vi "Read Locale.vi"(11 "MsgSerializer":refnum<class "MsgSerializer.lvclass">) -> (2 "Locale":string, 3 "MsgSerializer":refnum<class "MsgSerializer.lvclass">)   [LabVIEW 2013, in "Caraya.lvlib" / "MsgSerializer.lvclass"]
uses:
  MsgSerializer/MsgSerializer.lvclass
  MsgSerializer/MsgSerializer.lvclass/MsgSerializer.ctl
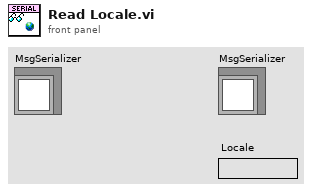
[diagram p1: front panel]
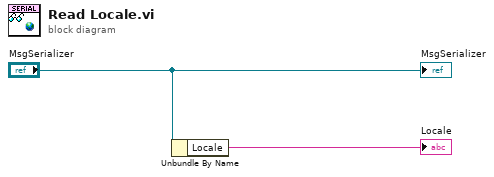
[diagram p0: block diagram]
diagram:
  n1 = Unbundle By Name("MsgSerializer") -> ("Locale"=→"Locale":string)
  "MsgSerializer" <- "MsgSerializer"
